vi "test json to variant float.vi"(8 "error in (no error)":errorcluster) -> (0 "error out":errorcluster)   [LabVIEW 2019, in "labview_json_tests.lvlib"]
uses:
  labview_json_tests.lvlib
  lib/labview_json.lvlib
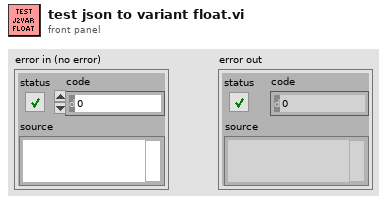
[diagram p1: front panel]
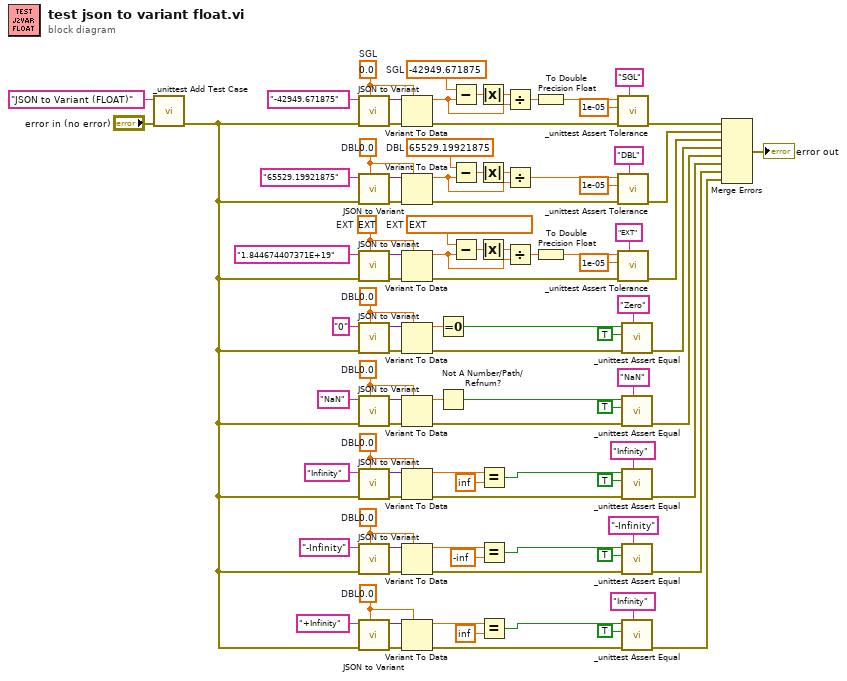
[diagram p0: block diagram]
diagram:
  w6 = 0.0  # DBL
  w17 = 0.0  # DBL
  w31 = 0.0  # DBL
  w39 = 0.0  # DBL
  w51 = 0.0  # DBL
  w64 = ext 1.844674407371e+19  # EXT
  w65 = ext 0.0  # EXT
  w76 = 65529.19921875  # DBL
  w75 = 0.0  # DBL
  w89 = sgl -42949.67  # SGL
  w90 = sgl 0.0  # SGL
  n1 = call "_unittest Add Test Case.vi"("error in (no error)"="error in (no error)", "Test Case"="JSON to Variant (FLOAT)") -> ("error out"=w2:errorcluster)  [unwired: 9 in]
  n2 = call "JSON to Variant.vi"("Variant Type"=w90, "error in (no error)"=w2, "JSON"="-42949.671875") -> ("error out"=w94:errorcluster, "Variant out"=w91:variant)  [unwired: 7 in]
  n3 = call "JSON to Variant.vi"("Variant Type"=w75, "error in (no error)"=w2, "JSON"="65529.19921875") -> ("error out"=w72:errorcluster, "Variant out"=w74:variant)  [unwired: 7 in]
  n4 = call "JSON to Variant.vi"("Variant Type"=w65, "error in (no error)"=w2, "JSON"="1.844674407371E+19") -> ("error out"=w68:errorcluster, "Variant out"=w66:variant)  [unwired: 7 in]
  n5 = call "JSON to Variant.vi"("Variant Type"=w51, "error in (no error)"=w2, "JSON"="0") -> ("error out"=w53:errorcluster, "Variant out"=w52:variant)  [unwired: 7 in]
  n6 = call "JSON to Variant.vi"("Variant Type"=w39, "error in (no error)"=w2, "JSON"="NaN") -> ("error out"=w37:errorcluster, "Variant out"=w38:variant)  [unwired: 7 in]
  n7 = call "JSON to Variant.vi"("Variant Type"=w31, "error in (no error)"=w2, "JSON"="Infinity") -> ("error out"=w33:errorcluster, "Variant out"=w32:variant)  [unwired: 7 in]
  n8 = call "JSON to Variant.vi"("Variant Type"=w17, "error in (no error)"=w2, "JSON"="-Infinity") -> ("error out"=w15:errorcluster, "Variant out"=w16:variant)  [unwired: 7 in]
  n9 = call "JSON to Variant.vi"("Variant Type"=w6, "error in (no error)"=w2, "JSON"="+Infinity") -> ("error out"=w4:errorcluster, "Variant out"=w5:variant)  [unwired: 7 in]
  n10 = Variant To Data(error in=w94, type=w90, Variant=w91) -> (data=w86:sgl, error out=w92:errorcluster)
  n11 = Variant To Data(error in=w72, type=w75, Variant=w74) -> (data=w79:dbl, error out=w73:errorcluster)
  n12 = Variant To Data(error in=w68, type=w65, Variant=w66) -> (data=w61:ext, error out=w67:errorcluster)
  n13 = Variant To Data(error in=w53, type=w51, Variant=w52) -> (data=w50:dbl, error out=w49:errorcluster)
  n14 = Variant To Data(error in=w37, type=w39, Variant=w38) -> (data=w40:dbl, error out=w41:errorcluster)
  n15 = Variant To Data(error in=w33, type=w31, Variant=w32) -> (data=w26:dbl, error out=w30:errorcluster)
  n16 = Variant To Data(error in=w15, type=w17, Variant=w16) -> (data=w21:dbl, error out=w18:errorcluster)
  n17 = Variant To Data(error in=w4, type=w6, Variant=w5) -> (data=w10:dbl, error out=w7:errorcluster)
  n18 = Equal To 0?(x=w50) -> (x = 0?=w46:bool)
  n19 = Not A Number/Path/Refnum?(number/path/refnum=w40) -> (NaN/Path/Refnum?=w43:bool)
  n20 = Subtract(x=w89, y=w86) -> (x-y=w88:sgl)
  n21 = Subtract(x=w76, y=w79) -> (x-y=w77:dbl)
  n22 = Subtract(x=w64, y=w61) -> (x-y=w63:ext)
  n23 = Absolute Value(x=w88) -> (abs(x)=w87:sgl)
  n24 = Absolute Value(x=w77) -> (abs(x)=w78:dbl)
  n25 = Absolute Value(x=w63) -> (abs(x)=w62:ext)
  n26 = Equal?(x=w26, y=inf) -> (x = y?=w25:bool)
  n27 = Equal?(x=w21, y=-inf) -> (x = y?=w22:bool)
  n28 = Equal?(x=w10, y=inf) -> (x = y?=w11:bool)
  n29 = Divide(x=w87, y=w86) -> (x/y=w85:sgl)
  n30 = Divide(x=w78, y=w79) -> (x/y=w80:dbl)
  n31 = Divide(x=w62, y=w61) -> (x/y=w60:ext)
  n32 = To Double Precision Float(number=w85) -> (double precision float=w56:dbl)
  n33 = To Double Precision Float(number=w60) -> (double precision float=w57:dbl)
  n34 = call "_unittest Assert Tolerance.vi"("Message"="SGL", "error in (no error)"=w92, "Tollerance (1E-5)"=1e-05, "Actual Value"=w56) -> ("error out"=w93:errorcluster)  [unwired: 7 in]
  n35 = call "_unittest Assert Tolerance.vi"("Message"="DBL", "error in (no error)"=w73, "Tollerance (1E-5)"=1e-05, "Actual Value"=w80) -> ("error out"=w70:errorcluster)  [unwired: 7 in]
  n36 = call "_unittest Assert Tolerance.vi"("Message"="EXT", "error in (no error)"=w67, "Tollerance (1E-5)"=1e-05, "Actual Value"=w57) -> ("error out"=w55:errorcluster)  [unwired: 7 in]
  n37 = call "_unittest Assert Equal.vi"("Message"="Zero", "error in (no error)"=w49, "Expected Value"=TRUE, "Actual Value"=w46) -> ("error out"=w48:errorcluster)  [unwired: 7 in]
  n38 = call "_unittest Assert Equal.vi"("Message"="NaN", "error in (no error)"=w41, "Expected Value"=TRUE, "Actual Value"=w43) -> ("error out"=w35:errorcluster)  [unwired: 7 in]
  n39 = call "_unittest Assert Equal.vi"("Message"="Infinity", "error in (no error)"=w30, "Expected Value"=TRUE, "Actual Value"=w25) -> ("error out"=w27:errorcluster)  [unwired: 7 in]
  n40 = call "_unittest Assert Equal.vi"("Message"="-Infinity", "error in (no error)"=w18, "Expected Value"=TRUE, "Actual Value"=w22) -> ("error out"=w13:errorcluster)  [unwired: 7 in]
  n41 = call "_unittest Assert Equal.vi"("Message"="Infinity", "error in (no error)"=w7, "Expected Value"=TRUE, "Actual Value"=w11) -> ("error out"=w1:errorcluster)  [unwired: 7 in]
  n42 = Merge Errors(w93, w70, w55, w48, w35, w27, w13, w1) -> (→"error out":errorcluster)
